vi "svx_Colormap Display from Cursor.vi"(8 "State":T1={"RefQueue"=refnum, "Properties/Undo"=refnum, "Bound"={"Width"=0, "Height"=0}, "Plot Area:Colors"={"FG Color"=11776947, "BG Color"=0}, "scale legend visible?"=FALSE, "graph palette visible?"=FALSE, "cursor palette visible?"=FALSE, "Ignore Array"=TRUE, "Smooth Update"=FALSE, "Z Scale"={"Z Scale.Scale Fit"=2, "Z Scale.Name Label.Text"="Amplitude", "Z Scale.Interpolate Color"=TRUE, "Visible"=TRUE, "Label Visible"=TRUE, "format string"="%#.2g", "Z Scale.Range"={"Minimum"=0.0, "Maximum"=500.0}}, "X Scale"={"X Scale.Scale Fit"=2, "X Scale.Offset and Multiplier"={"Offset"=0.0, "Multiplier"=1.0}, "X Scale.Name Label.Text"="Time", "X Scale.Range"={"Minimum"=0.0, "Maximum"=10.0}, "Visible"=TRUE, "Label Visible"=TRUE, "format string"="%#.2g"}, "Y Scale"={"Y Scale.Scale Fit"=2, "Y Scale.Offset and Multiplier"={"Offset"=0.0, "Multiplier"=1.0}, "Y Scale.Name Label.Text"="Frequency", "Y Scale.Range"={"Minimum"=0.0, "Maximum"=500.0}, "Visible"=TRUE, "Label Visible"=TRUE, "format string"="%#.2g"}, "Annotation List"=[], "Cursor List"=[], "Display Frequency Lines"=TRUE, "Display Order Lines"=TRUE, "Display Order text"=TRUE, "Display Frequency text"=TRUE, "Order Lineproperty"={"Line"={"Width"=1, "Style"=enum."Dash"}, "color"=0}, "Order Textproperty"={"Test size"=11, "color"=16777222, "background"=16777216}, "Orders"=[], "Frequency"=[], "Frequency Lineproperty"={"Line"={"Width"=1, "Style"=enum."Dash"}, "color"=0}, "Frequency Textproperty"={"Test size"=11, "color"=16777222, "background"=16777216}, "Display Order from Cursor"=FALSE, "Display Freq from Cursor"=FALSE, "Active Cursor"=0, "Selected Cursors"=[], "Cursor Move"=refnum, "Scale Range Change"=refnum}, 9 "Data In":T2 {"Y scale"."multiplier" format="%.2f"; "Y scale"."offset" format="%.2f"; "X scale"."multiplier" format="%.2f"; "X scale"."offset" format="%.2f"; "spectral map" format="%.2f"}, 10 "new picture in":picture, 11 "Color Map in":refnum<vi>) -> (2 "new picture out":picture, 3 "Color Map out":refnum<vi>)   [LabVIEW 2017, in "SVX Colormap.xctl"]
uses:
  <vilib>/addons/_XControls/Colormap/SVX Colormap.xctl
  <vilib>/addons/_XControls/Colormap/subVIs/svx_Colormap Data.ctl
  <vilib>/addons/_XControls/Colormap/subVIs/svx_Colormap State.ctl
  <vilib>/addons/_XControls/Colormap/TypeDef/svx_Colormap_InnerState.ctl
  <vilib>/addons/_XControls/Colormap/TypeDef/svx_Colormap_Event.ctl
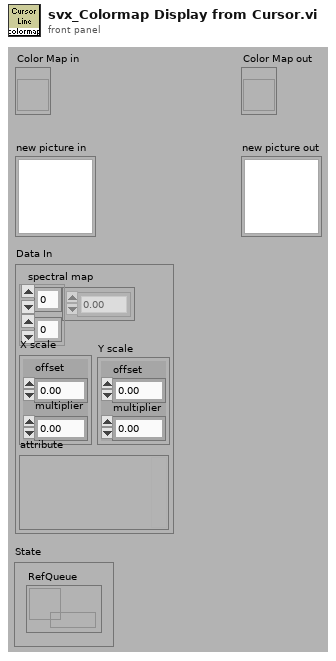
[diagram p1: front panel]
types:
  T1 = typedef "SVX Colormap.xctl/svx_Colormap State.ctl" = cluster{"RefQueue":refnum<queue>, "Properties/Undo":refnum<queue>, "Bound":cluster{"Width":u32, "Height":u32}, "Plot Area:Colors":cluster{"FG Color":u32, "BG Color":u32}, "scale legend visible?":bool, "graph palette visible?":bool, "cursor palette visible?":bool, "Ignore Array":bool, "Smooth Update":bool, "Z Scale":cluster{"Z Scale.Scale Fit":u8, "Z Scale.Name Label.Text":string, "Z Scale.Interpolate Color":bool, "Visible":bool, "Label Visible":bool, "format string":string, "Z Scale.Range":cluster{"Minimum":dbl, "Maximum":dbl}}, "X Scale":cluster{"X Scale.Scale Fit":u8, "X Scale.Offset and Multiplier":cluster{"Offset":dbl, "Multiplier":dbl}, "X Scale.Name Label.Text":string, "X Scale.Range":cluster{"Minimum":dbl, "Maximum":dbl}, "Visible":bool, "Label Visible":bool, "format string":string}, "Y Scale":cluster{"Y Scale.Scale Fit":u8, "Y Scale.Offset and Multiplier":cluster{"Offset":dbl, "Multiplier":dbl}, "Y Scale.Name Label.Text":string, "Y Scale.Range":cluster{"Minimum":dbl, "Maximum":dbl}, "Visible":bool, "Label Visible":bool, "format string":string}, "Annotation List":cluster{"Name":string, "Color":u32, "Style":u8, "Point Style":u8, "Name Visible":bool, "Allow Drag":bool, "Annotation Mode":u32, "Plot":i32, "Index":i32, "Position":cluster{"X":dbl, "Y":dbl}, "X Scale":u32, "Y Scale":u32, "Show Arrow":bool, "Lock Name":bool, "Plot Area":i32, "Label Offset":cluster{"X":dbl, "Y":dbl}}[], "Cursor List":cluster{"Name":string, "Color":u32, "Style":u8, "Point Style":u8, "Name Visible":bool, "Allow Drag":bool, "Cursor Mode":u32, "Plot":i32, "Index":i32, "Position":cluster{"X":dbl, "Y":dbl}, "X Scale":u32, "Y Scale":u32, "Watch Plots":i32[], "Watch All Plots":bool, "Plot Area":i32, "Label Offset":cluster{"X":dbl, "Y":dbl}}[], "Display Frequency Lines":bool, "Display Order Lines":bool, "Display Order text":bool, "Display Frequency text":bool, "Order Lineproperty":cluster{"Line":cluster{"Width":u16, "Style":enum32{"Solid", "Dash", "Dot", "DashDot", "DashDotDot"}}, "color":u32}, "Order Textproperty":cluster{"Test size":i16, "color":u32, "background":u32}, "Orders":dbl[], "Frequency":dbl[], "Frequency Lineproperty":cluster{"Line":cluster{"Width":u16, "Style":enum32{"Solid", "Dash", "Dot", "DashDot", "DashDotDot"}}, "color":u32}, "Frequency Textproperty":cluster{"Test size":i16, "color":u32, "background":u32}, "Display Order from Cursor":bool, "Display Freq from Cursor":bool, "Active Cursor":u32, "Selected Cursors":u32[], "Cursor Move":refnum<user-event>, "Scale Range Change":refnum<user-event>}
  T2 = typedef "SVX Colormap.xctl/svx_Colormap Data.ctl" = cluster{"spectral map":dbl[][], "X scale":cluster{"offset":dbl, "multiplier":dbl}, "Y scale":cluster{"offset":dbl, "multiplier":dbl}, "attribute":variant}
  T3 = enum16{"Frequency-Time", "Time-Frequency", "Order-Time", "Time-Order", "Frequency-RPM", "RPM-Frequency", "Order-RPM", "RPM-Order"}
  T4 = cluster{"Line":cluster{"Width":u16, "Style":enum32{"Solid", "Dash", "Dot", "DashDot", "DashDotDot"}}, "color":u32}
  T5 = cluster{"Test size":i16, "color":u32, "background":u32}
  T6 = typedef "LVCursorListTypeDef.ctl" = cluster{"Name":string, "Color":u32, "Style":u8, "Point Style":u8, "Name Visible":bool, "Allow Drag":bool, "Cursor Mode":u32, "Plot":i32, "Index":i32, "Position":cluster{"X":dbl, "Y":dbl}, "X Scale":u32, "Y Scale":u32, "Watch Plots":i32[], "Watch All Plots":bool, "Plot Area":i32, "Label Offset":cluster{"X":dbl, "Y":dbl}}[]
  T7 = cluster{"Name":string, "Color":u32, "Style":u8, "Point Style":u8, "Name Visible":bool, "Allow Drag":bool, "Cursor Mode":u32, "Plot":i32, "Index":i32, "Position":cluster{"X":dbl, "Y":dbl}, "X Scale":u32, "Y Scale":u32, "Watch Plots":i32[], "Watch All Plots":bool, "Plot Area":i32, "Label Offset":cluster{"X":dbl, "Y":dbl}}
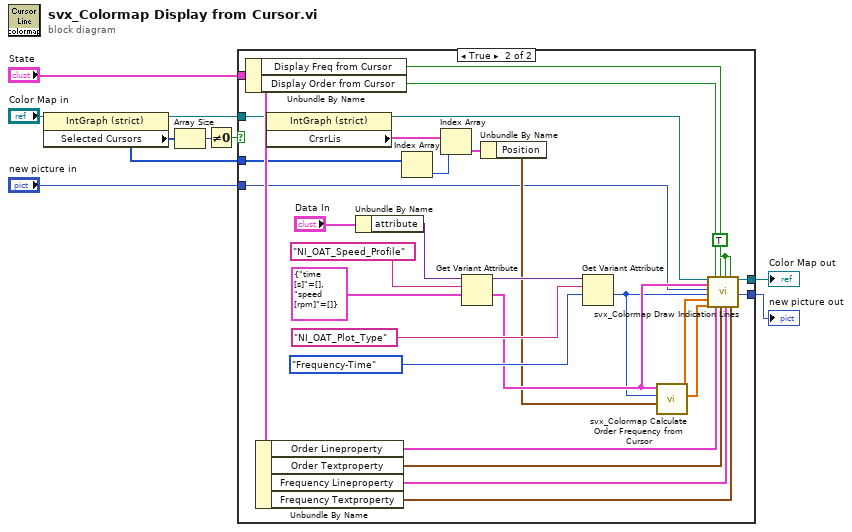
[diagram p0: block diagram]
diagram:
  n1 = property class="IntGraph (strict)"(reference="Color Map in") -> (reference out=w2:refnum<vi>, "Selected Cursors"=w1:u32[])  [unwired: 1 in, 1 out]
  n2 = Array Size(array=w1) -> (size(s)=w8:i32)
  n3 = Not Equal To 0?(x=w8) -> (x != 0?=w7:bool)
  n4 = case shown="True" w7 {
    tunnel: [w11 w40] -> w9
    tunnel: w2 -> [w11 w15]
    tunnel: "State" -> [_ w22]
    tunnel: [w10 w17] -> w5
    tunnel: "new picture in" -> [w10 w16]
    tunnel: w1 -> [_ w13]
    frame False {
    }
    frame True {
      w32 = TRUE ("Ordertext")
      n5 = Unbundle By Name(w22) -> ("Display Freq from Cursor"=w30:bool, "Display Order from Cursor"=w31:bool)
      n6 = Unbundle By Name(w22) -> ("Order Lineproperty"=w21:T4, "Order Textproperty"=w20:T5, "Frequency Lineproperty"=w19:T4, "Frequency Textproperty"=w18:T5)
      n7 = property class="IntGraph (strict)"(reference=w15) -> (reference out=w12:refnum<vi>, "CrsrLis"=w14:T6)  [unwired: 1 in, 1 out]
      n8 = Unbundle By Name("Data In") -> ("attribute"=w39:variant)
      n9 = Index Array(array=w13) -> (element=w23:u32)  [unwired: 1 in]
      n10 = Index Array(array=w14, index=w23) -> (element=w25:T7)
      n11 = Get Variant Attribute(Variant=w39, name="NI_OAT_Speed_Profile", default value (empty Variant)=cluster{"time [s]":dbl[], "speed [rpm]":dbl[]} {"time [s]"=[], "speed [rpm]"=[]} ("speed profile")) -> (duplicate Variant=w38:variant, value=w29:cluster{"time [s]":dbl[], "speed [rpm]":dbl[]})  [unwired: 1 in, 2 out]
      n12 = Unbundle By Name(w25) -> ("Position"=w24:cluster{"X":dbl, "Y":dbl})
      n13 = Get Variant Attribute(Variant=w38, name="NI_OAT_Plot_Type", default value (empty Variant)=T3."Frequency-Time" ("plot type")) -> (value=w28:T3)  [unwired: 1 in, 3 out]
      n14 = call <vilib>:"svx_Colormap Calculate Order Frequency from Cursor.vi"("CursLoc"=w24, "plot type"=w28, "speed profile"=w29) -> ("Order type"=w26:dbl[], "Frequency type"=w27:dbl[])  [unwired: 7 in]
      n15 = call <vilib>:"svx_Colormap Draw Indication Lines.vi"("color map ref in"=w12, "speed profile"=w29, "new picture 2"=w16, "plot type"=w28, "Frequency type"=w27, "Order type"=w26, "Display Order"=w31, "orderline setting"=w21, "Display Frequency"=w30, "ordertext setting"=w20, "Ordertext"=w32, "frequencyline setting"=w19, "Frequencytext"=w32, "frequencytext setting"=w18) -> ("color map ref out"=w40:refnum<vi>, "Plot Images:Front"=w17:picture)  [unwired: 4 in]
    }
  }
  "Color Map out" <- w9
  "new picture out" <- w5
